vi "writeToXML.vi"(8 "error in (no error)":errorcluster, 10 "Class label":string, 11 "TCSGuiderStatus in":refnum<class "TCSGuideStatus.lvclass">) -> (0 "error out":errorcluster, 2 "outputXMLString":string, 3 "TCSGuiderStatus out":refnum<class "TCSGuideStatus.lvclass">)   [LabVIEW 2014, in "TCSDataDefinitions.lvlib" / "TCSGuiderStatus.lvlib" / "TCSGuideStatus.lvclass"]
uses:
  TCSGuideStatus.lvclass
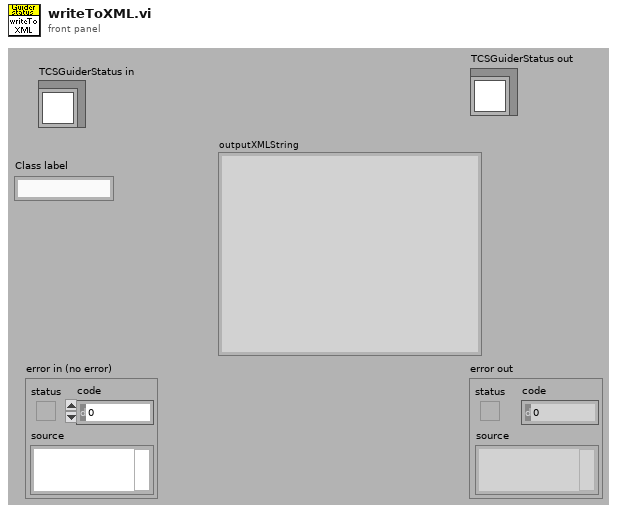
[diagram p1: front panel]
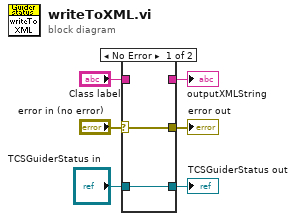
[diagram p0: block diagram]
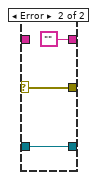
[diagram p2: hidden frame]
diagram:
  n1 = case shown="No Error" "error in (no error)" {
    selector: "error in (no error)" -> [w7 w11]
    tunnel: [w7 w11] -> w5
    tunnel: [w8 w10] -> w4
    tunnel: "TCSGuiderStatus in" -> [w8 w10]
    tunnel: [_ ""] -> w3
    tunnel: "Class label" -> [_ _]
    frame No Error {
    }
    frame Error {
    }
  }
  "error out" <- w5
  "TCSGuiderStatus out" <- w4
  "outputXMLString" <- w3
